vi "Fix Toolbar window up.vi"(1 "Error In (no error)":errorcluster, 2 "Toolbar Refnum":refnum<vi>, 3 "Parent Vi":refnum<vi>) -> (0 "error out":errorcluster)   [LabVIEW 2012]
uses:
  Toolbar.xctl
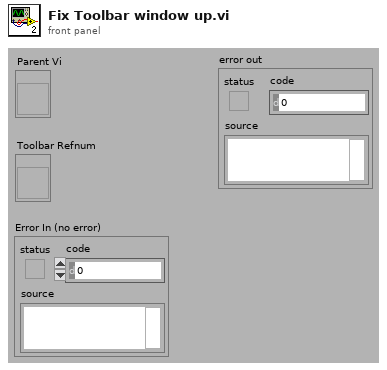
[diagram p1: front panel]
types:
  T1 = typedef "LVRectTypeDef.ctl" = cluster{"Left":i16, "Top":i16, "Right":i16, "Bottom":i16}
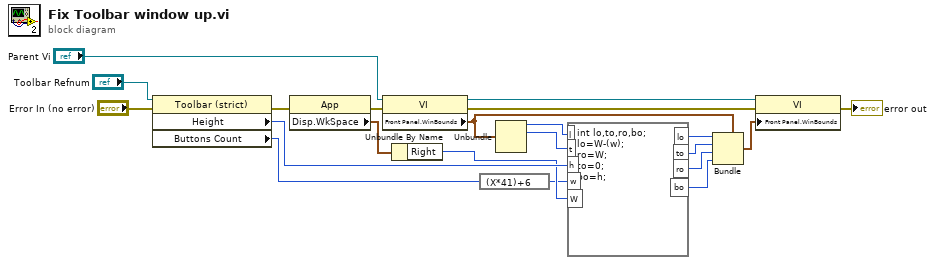
[diagram p0: block diagram]
diagram:
  n1 = property on="Property Node" class="Toolbar (strict)"(reference="Toolbar Refnum", error in="Error In (no error)") -> (error out=w17:errorcluster, "Height"=w18:u32, "Buttons Count"=w19:i32)  [unwired: 1 out]
  n2 = property class="App"(error in=w17) -> (error out=w5:errorcluster, "Disp.WkSpace"=w4:T1)  [unwired: 1 in, 1 out]
  n3 = property class="VI"(reference="Parent Vi", error in=w5) -> (reference out=w15:refnum<vi>, error out=w16:errorcluster, "Front Panel.WinBounds"=w13:T1)
  n4 = Unbundle By Name(w4) -> ("Right"=w8:i16)
  n5 = expression code="(X*41)+6"(w19) -> (w1:i32)
  n6 = Unbundle(w13) -> ("Left"=w6:i16, "Top"=w7:i16)  [unwired: 2 out]
  n7 = formula code="int lo,to,ro,bo;\nlo=W-(w);\nro=W;\nto=0;\nbo=h;"("l"=w6, "t"=w7, "h"=w18, "w"=w1, "W"=w8) -> ("lo"=w9:i32, "to"=w10:i32, "ro"=w11:i32, "bo"=w12:i32)
  n8 = Bundle(cluster=w13, "Left"=w9, "Top"=w10, "Right"=w11, "Bottom"=w12) -> (w14:T1)
  n9 = property class="VI"(reference=w15, error in=w16, "Front Panel.WinBounds"=w14) -> (error out=→"error out":errorcluster)  [unwired: 1 out]
